vi "to_local_coords.vi"(8 "error in":errorcluster, 9 "orientation":cluster{"pitch":dbl, "roll":dbl, "yaw":dbl}, 10 "offset":cluster{"x":dbl, "y":dbl, "z":dbl}, 11 "global":cluster{"x":dbl, "y":dbl, "z":dbl}) -> (0 "error out":errorcluster, 3 "local":cluster{"x":dbl, "y":dbl, "z":dbl})   [LabVIEW 2011, in "gVision.lvlib"]
uses:
  gVision.lvlib
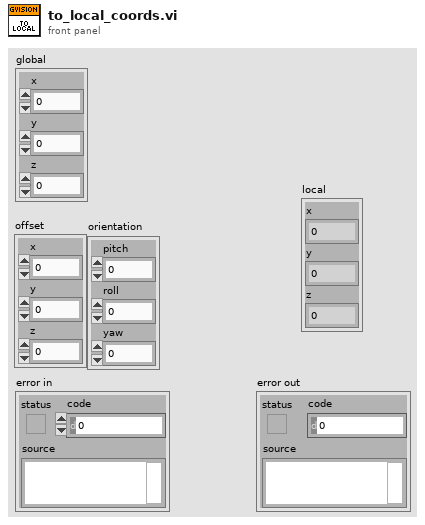
[diagram p1: front panel]
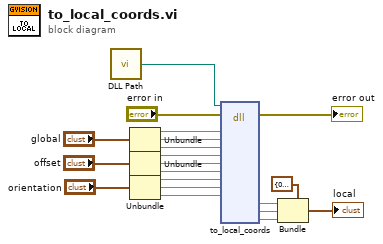
[diagram p0: block diagram]
diagram:
  n1 = call "DLL Path.vi"() -> ("DLL Path"=w20:path)  [unwired: 5 in]
  n2 = Unbundle("global") -> ("x"=w16:dbl, "y"=w15:dbl, "z"=w14:dbl)
  n3 = Unbundle("offset") -> ("x"=w12:dbl, "y"=w11:dbl, "z"=w10:dbl)
  n4 = Unbundle("orientation") -> ("pitch"=w8:dbl, "roll"=w7:dbl, "yaw"=w6:dbl)
  n5 = dll-call lib="?" fn="to_local_coords"(path in=w20, error in="error in", "global_x"=w16, "global_y"=w15, "global_z"=w14, "offset_x"=w12, "offset_y"=w11, "offset_z"=w10, "pitch"=w8, "roll"=w7, "yaw"=w6) -> (error out=→"error out":errorcluster, "local_x"=w4:dbl, "local_y"=w3:dbl, "local_z"=w2:dbl)  [unwired: 14 in, 1 out]
  n6 = Bundle(cluster=cluster{"x":dbl, "y":dbl, "z":dbl} {"x"=0.0, "y"=0.0, "z"=0.0} ("local 2"), "x"=w4, "y"=w3, "z"=w2) -> (→"local":cluster{"x":dbl, "y":dbl, "z":dbl})
